vi "Write Map.vi"(8 "error in":errorcluster, 10 "map from values indexes to RT info indexes":T1, 11 "Ballard ARINC-429 Tx execution unit in":refnum<class "Tx Acyclic Labels Execution Unit.lvclass">) -> (0 "error out":errorcluster, 3 "Ballard ARINC-429 Tx execution unit out":refnum<class "Tx Acyclic Labels Execution Unit.lvclass">)   [LabVIEW 2020, in "Ballard ARINC 429 Engine.lvlib" / "Implementation.lvlib" / "Tx Acyclic Labels Execution Unit.lvclass"]
uses:
  Tx Acyclic Labels Execution Unit.lvclass
  Shared/Map of Values Indexes to Channel and Label Indexes.ctl
  Tx Acyclic Labels Execution Unit.lvclass/Tx Acyclic Labels Execution Unit.ctl
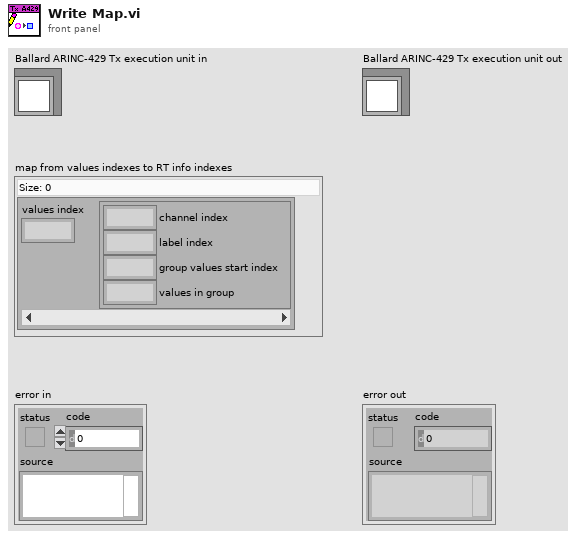
[diagram p1: front panel]
types:
  T1 = typedef "Map of Values Indexes to Channel and Label Indexes.ctl" = map{i32, cluster{"channel index":i32, "label index":i32, "group values start index":i32, "values in group":i32}}
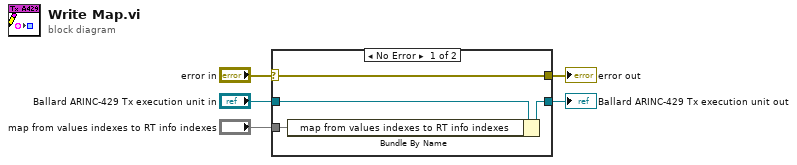
[diagram p0: block diagram]
diagram:
  n1 = case shown="No Error" "error in" {
    selector: "error in" -> [w9 w10]
    tunnel: [w9 w10] -> w4
    tunnel: [w6 w11] -> w2
    tunnel: "Ballard ARINC-429 Tx execution unit in" -> [w8 w11]
    tunnel: "map from values indexes to RT info indexes" -> [w7 _]
    frame No Error {
      n2 = Bundle By Name(cluster=w8, "map from values indexes to RT info indexes"=w7) -> (w6:refnum<class "Tx Acyclic Labels Execution Unit.lvclass">)
    }
    frame Error {
    }
  }
  "error out" <- w4
  "Ballard ARINC-429 Tx execution unit out" <- w2
